vi "counter read write.vi"(3 "OK :T":bool, 5 "NG Part":i32, 7 "OK Part":i32, 8 "Action":enum16{"read", "write"}(ring), 10 "Model No.":string, 11 "Count Path":path) -> (0 "NG Part Out":i32, 1 "OK Part Out":i32)   [LabVIEW 2015]
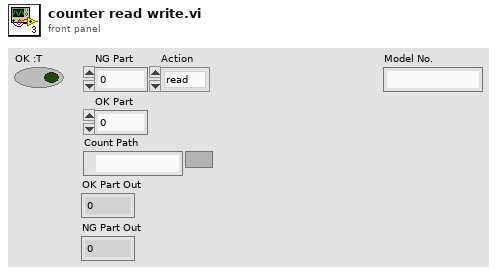
[diagram p1: front panel]
types:
  T1 = enum16{"open", "replace", "create", "open or create", "replace or create", "replace or create with confirmation"}
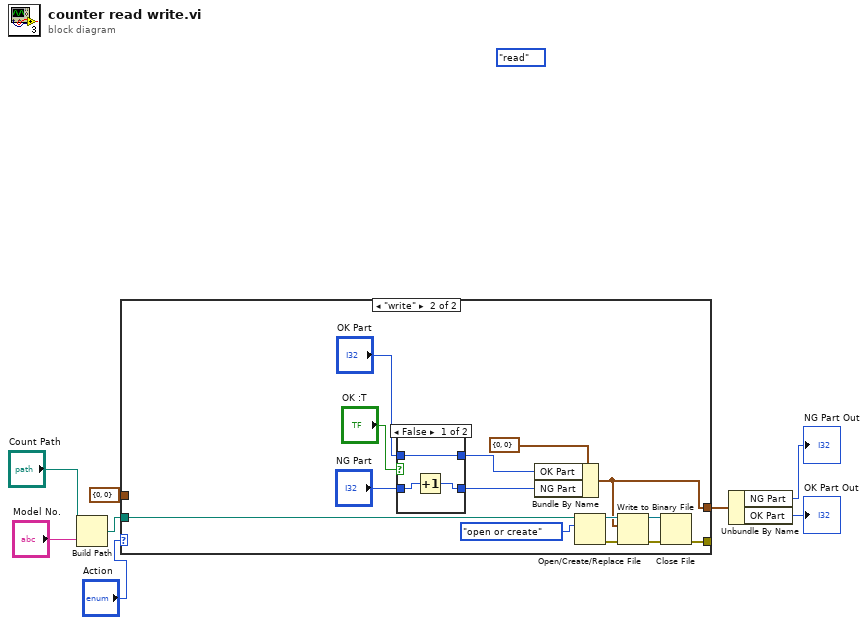
[diagram p0: block diagram]
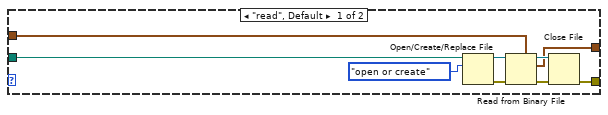
[diagram p2: hidden frame]
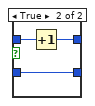
[diagram p3: hidden frame]
diagram:
  (unwired) enum16{"read", "write"}."read"
  n1 = Build Path(base path="Count Path", name or relative path="Model No.") -> (appended path=w8:path)
  n2 = case shown="\"write\"" "Action" {
    tunnel: w8 -> [w12 w28]
    tunnel: cluster{"OK Part":i32, "NG Part":i32} {"OK Part"=0, "NG Part"=0} ("Cluster") -> [w11 _]
    tunnel: [w10 w24] -> w3
    tunnel: [w9 w18] -> _
    frame "read", Default {
      n3 = Open/Create/Replace File(file path (use dialog)=w12, operation (0:open)=T1."open or create") -> (refnum out=w17:refnum<file>, error out=w14:errorcluster)  [unwired: 4 in, 1 out]
      n4 = Read from Binary File(5:w11, 8:w14, 11:w17) -> (0:w13:errorcluster, 2:w10:cluster{"OK Part":i32, "NG Part":i32}, 3:w16:refnum<file>)  [unwired: 3 in, 1 out]
      n5 = Close File(refnum=w16, error in=w13) -> (error out=w9:errorcluster)  [unwired: 1 out]
    }
    frame "write" {
      n6 = case shown="False" "OK :T" {
        tunnel: [w34 w35] -> w22
        tunnel: "OK Part" -> [w34 w37]
        tunnel: [w32 w36] -> w20
        tunnel: "NG Part" -> [w33 w36]
        frame False {
          n7 = Increment(x=w33) -> (x+1=w32:i32)
        }
        frame True {
          n8 = Increment(x=w37) -> (x+1=w35:i32)
        }
      }
      n9 = Bundle By Name(cluster=cluster{"OK Part":i32, "NG Part":i32} {"OK Part"=0, "NG Part"=0} ("Cluster 2"), "OK Part"=w22, "NG Part"=w20) -> (w24:cluster{"OK Part":i32, "NG Part":i32})
      n10 = Open/Create/Replace File(file path (use dialog)=w28, operation (0:open)=T1."open or create") -> (refnum out=w31:refnum<file>, error out=w27:errorcluster)  [unwired: 4 in, 1 out]
      n11 = Write to Binary File(file (use dialog)=w31, data=w24, error in=w27) -> (refnum out=w30:refnum<file>, error out=w26:errorcluster)  [unwired: 3 in, 1 out]
      n12 = Close File(refnum=w30, error in=w26) -> (error out=w18:errorcluster)  [unwired: 1 out]
    }
  }
  n13 = Unbundle By Name(w3) -> ("NG Part"=→"NG Part Out":i32, "OK Part"=→"OK Part Out":i32)
